vi "ESP301_Read_Double_Position.vi"(11 "COM_PORT":string="COM12") -> (0 "MD 2":bool, 1 "errstring 6":string, 2 "errstring 3":string, 3 "MD":bool, 4 "Motor_status 2":bool, 5 "Motor_status":bool, 6 "Position 2":dbl, 7 "Position":dbl)   [LabVIEW 2019]
uses:
  Newport.ESP301.CommandInterface
panel:
  out "MD 3":i32
  out "errstring 5":string
  out "MO_Get 2":i32
  out "TP 2":i32
  out "errstring 4":string
  out "MD":i32
  out "errstring 2":string
  out "MO_Get":i32
  out "TP":i32
  out "errstring":string
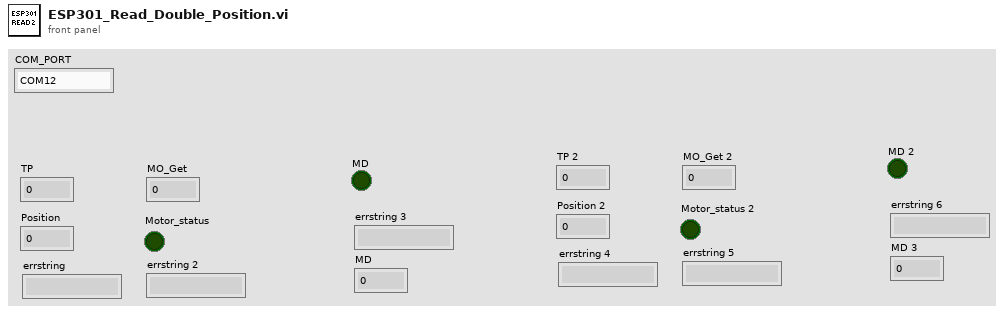
[diagram p1: front panel]
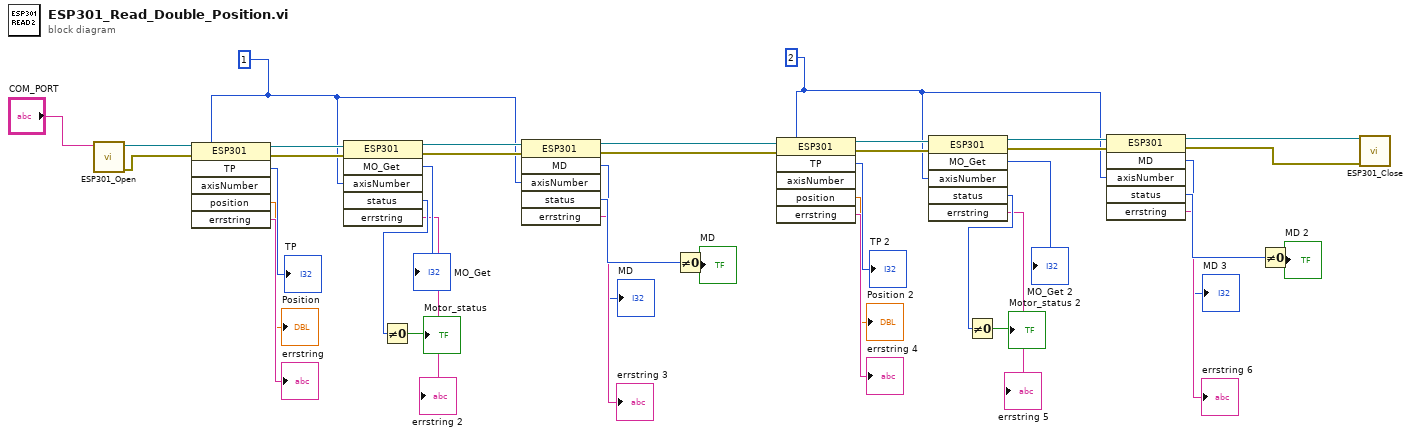
[diagram p0: block diagram]
diagram:
  w5 = 2
  w6 = 1
  n1 = call "ESP301_Open.vi"("strDeviceKey"="COM_PORT") -> ("sortie d'erreur"=w36:errorcluster, "référence en sortie"=w37:refnum<k24>)  [unwired: 9 in]
  n2 = invoke on="Nœud de méthode" class="ESP301" method="TP"(reference=w37, error in=w36, "axisNumber"=w6) -> (reference out=w39:refnum<k24>, error out=w38:errorcluster, "TP"=→"TP":i32, "position"=→"Position":dbl, "errstring"=→"errstring":string)  [unwired: 3 in, 1 out]
  n3 = invoke on="Nœud de méthode" class="ESP301" method="MO_Get"(reference=w39, error in=w38, "axisNumber"=w6) -> (reference out=w27:refnum<k24>, error out=w26:errorcluster, "MO_Get"=→"MO_Get":i32, "status"=w31:i32, "errstring"=→"errstring 2":string)  [unwired: 3 in, 1 out]
  n4 = Not Equal To 0?(x=w31) -> (x != 0?=→"Motor_status":bool)
  n5 = invoke on="Nœud de méthode" class="ESP301" method="MD"(reference=w27, error in=w26, "axisNumber"=w6) -> (reference out=w4:refnum<k24>, error out=w3:errorcluster, "MD"=→"MD":i32, "status"=w25:i32, "errstring"=→"errstring 3":string)  [unwired: 3 in, 1 out]
  n6 = Not Equal To 0?(x=w25) -> (x != 0?=→"MD":bool)
  n7 = invoke on="Nœud de méthode" class="ESP301" method="TP"(reference=w4, error in=w3, "axisNumber"=w5) -> (reference out=w21:refnum<k24>, error out=w20:errorcluster, "TP"=→"TP 2":i32, "position"=→"Position 2":dbl, "errstring"=→"errstring 4":string)  [unwired: 3 in, 1 out]
  n8 = invoke on="Nœud de méthode" class="ESP301" method="MO_Get"(reference=w21, error in=w20, "axisNumber"=w5) -> (reference out=w12:refnum<k24>, error out=w11:errorcluster, "MO_Get"=→"MO_Get 2":i32, "status"=w15:i32, "errstring"=→"errstring 5":string)  [unwired: 3 in, 1 out]
  n9 = Not Equal To 0?(x=w15) -> (x != 0?=→"Motor_status 2":bool)
  n10 = invoke on="Nœud de méthode" class="ESP301" method="MD"(reference=w12, error in=w11, "axisNumber"=w5) -> (reference out=w2:refnum<k24>, error out=w1:errorcluster, "MD"=→"MD 3":i32, "status"=w10:i32, "errstring"=→"errstring 6":string)  [unwired: 3 in, 1 out]
  n11 = Not Equal To 0?(x=w10) -> (x != 0?=→"MD 2":bool)
  n12 = call "ESP301_Close.vi"("entrée d'erreur (pas d'erreur)"=w1, "référence"=w2) -> ()  [unwired: 9 in, 1 out]
